vi "Extract_variable_double.vi"(2 "key":string, 3 "InputString":string) -> (0 "Output":dbl, 1 "outstring":string)   [LabVIEW 2011]
doc: "regular expression to parse value out of string in certain files such as Phillips Tiff files."
uses:
  <vilib>/regexp/Match Regular Expression.xnode
panel:
  out "error out":errorcluster
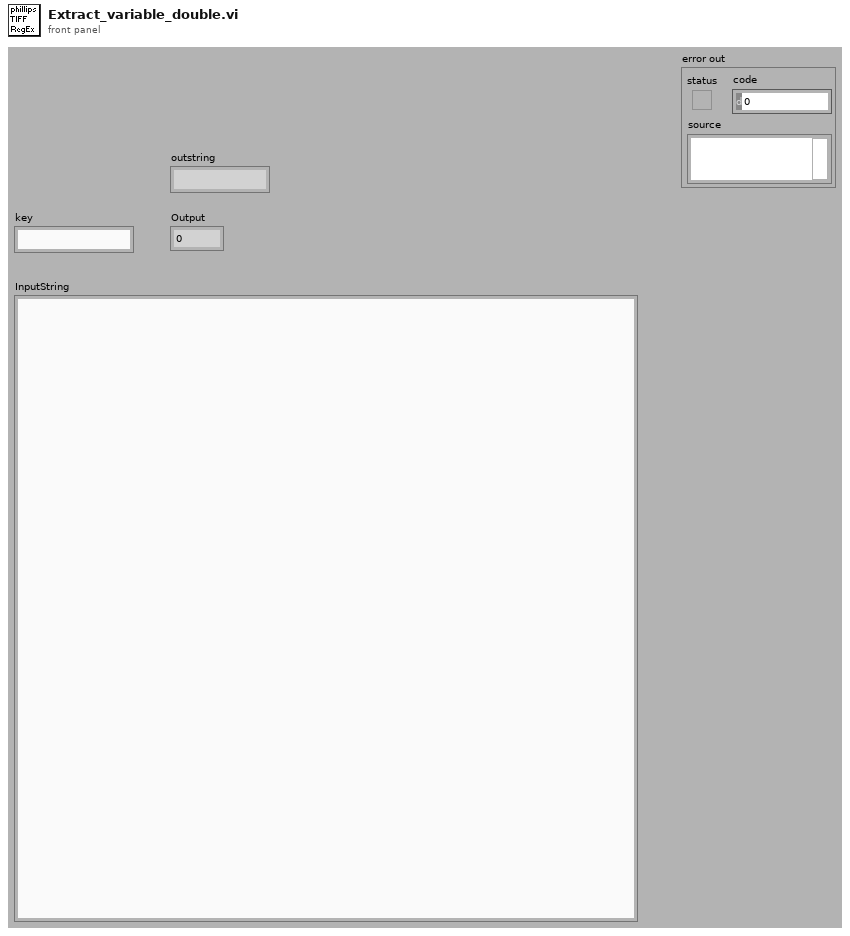
[diagram p1: front panel]
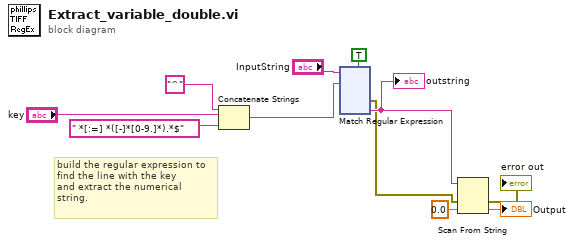
[diagram p0: block diagram]
diagram:
  # "build the regular expression to\nfind the line with the key \nand extract the numerical\nstring."
  n1 = Concatenate Strings("^" ("input string"), "key", " *[:=] *([-]*[0-9.]*).*$" ("input string")) -> (w11:string)
  n2 = xnode "Match Regular Expression"("input string"="InputString", "regular expression"=w11, "multiline? (F)"=TRUE) -> ("error out"=w2:errorcluster, "submatch 1"=w6:string)  [unwired: 2 in, 5 out]
  "outstring" <- w6
  n3 = Scan From String(input string=w6, error in=w2, default 1=0.0 ("default value 1")) -> (error out=→"error out":errorcluster, output 1=→"Output":dbl)  [unwired: 2 in, 2 out]
